vi "Unpack for gRPC.vi"(8 "error in":errorcluster, 9 "configuration / results":enum16{"Configuration", "Results"}(ring), 10 "any":T1, 11 "measurement plugin in":refnum<class "Automotive Vision.lvclass">) -> (0 "error out":errorcluster, 2 "data value":variant, 3 "measurement plugin out":refnum<class "Automotive Vision.lvclass">)   [LabVIEW 2025, in "Automotive Vision.lvclass"]
uses:
  Automotive Vision.lvclass
  <vilib>/gRPC/LabVIEW gRPC Library/Shared/Any.ctl
  C:/Program Files/National Instruments/LabVIEW 2025/vi.lib/Plug-In SDKs/Measurements/Measurement Plugin Service/Measurement Plugin Service.lvclass
  Measurement Configuration.ctl
  Measurement Results.ctl
  a521b266-ce99-437c-923d-067dcf1e07fd.vi
  3ecd018e-d556-4cbc-bc60-c4ba57204520.vi
  <vilib>/gRPC/LabVIEW gRPC Library/Server API/Translate Protobuf Error.vi
  <vilib>/AdvancedString/1D String Array to Delimited String.vi
  <vilib>/gRPC/LabVIEW gRPC Library/Server API/Server/Get Server DLL Path.vi
  <vilib>/Plug-In SDKs/Measurements/Measurement Plugin Service/Measurement Plugin Service.lvclass
  <vilib>/gRPC/LabVIEW gRPC Library/grpc-lvsupport-release.lvlib
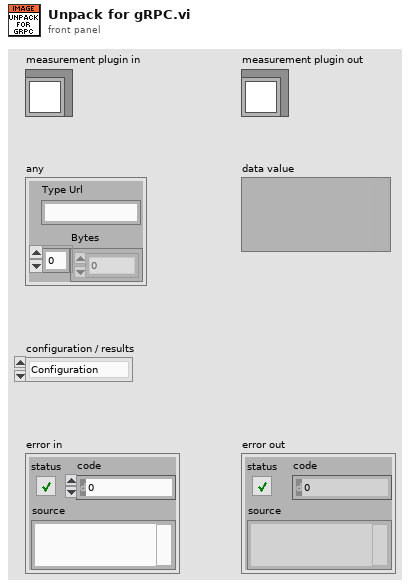
[diagram p1: front panel]
types:
  T1 = typedef "grpc-lvsupport-release.lvlib/Any.ctl" = cluster{"Type Url":string, "Bytes":u8[]}
  T2 = typedef "grpc-lvsupport-release.lvlib/grpcId.ctl" = u64
  T3 = typedef "Automotive Vision.lvclass/Measurement Configuration.ctl" = cluster{"SERIAL CHANNEL":string, "PATH TO CONFIGURATION SCRIPT":string, "REF. CLOCK  (Hz)":dbl, "POC SOURCE":u32, "CSI-2 DATA SOURCE":u32, "SI ACTIVE LANE CNT":u32, "PAYLOAD DATA TYPE":enum32{"Frame Start", "Frame End", "Line Start", "Line End", "End of Transmission", "Reserved 0", "Reserved 1", "Reserved 2", "Generic Short Packet 1", "Generic Short Packet 2", "Generic Short Packet 3", "Generic Short Packet 4", "Generic Short Packet 5", "Generic Short Packet 6", "Generic Short Packet 7", "Generic Short Packet 8", "Null", "Blanking Data", "Embedded 8-bit non Image Data", "Generic Long Packet 1", "Generic Long Packet 2", "Generic Long Packet 3", "Generic Long Packet 4", "Reserved 3", "YUV420 8-bit", "YUV420 10-bit", "Legacy YUV420 8-bit", "Reserved 4", "YUV420 8-bit Chroma Shifted", "YUV420 10-bit Chroma Shifted", "YUV422 8-bit", "YUV422 10-bit", "RGB444", "RGB555", "RGB565", "RGB666", "RGB888", "Reserved 5", "Reserved 6", "RAW 24", "RAW 6", "RAW 7", "RAW 8", "RAW 10", "RAW 12", "RAW 14", "RAW 16", "RAW 20", "User Defined 8-bit Data 1", "User Defined 8-bit Data 2", "User Defined 8-bit Data 3", "User Defined 8-bit Data 4", "User Defined 8-bit Data 5", "User Defined 8-bit Data 6", "User Defined 8-bit Data 7", "User Defined 8-bit Data 8", "USL Command", "Reserved 7", "Reserved 8", "Reserved 9", "Reserved 10", "Reserved 11", "Reserved 12", "LRTE EPD Spacer"}, "INTERPRETATION":u32, "VIRTUAL CHANNEL":u32, "PATTERN":u32, "ALGORITHM":u32, "RIO HANDLER":string, "AUTO. VISION DEVICE":u32, "SERIAL (SI) CHANNEL":u32, "BITFILE":string}
  T4 = typedef "Automotive Vision.lvclass/Measurement Results.ctl" = cluster{"ACQ. IN PROGRESS":bool, "IMAGE PIXEL DATA":u32[], "ACQ. DURATION (s)":dbl, "SOURCE RATE (fps)":dbl, "BYTES ACQUIRED":u64, "FRAME COUNT":u64, "POC VOLTAGE (V)":dbl, "POC CURRENT (A)":dbl, "ERROR":bool, "STATE MESSAGE":string, "IMAGE DATA":string, "OOB gRPC Port":i32, "HEIGHT":u64, "WIDTH":u64}
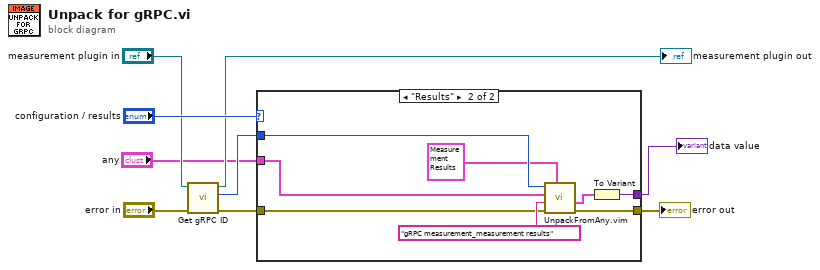
[diagram p0: block diagram]
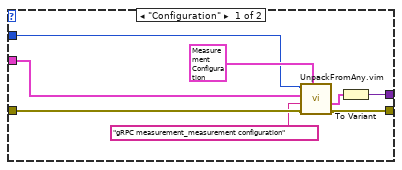
[diagram p2: hidden frame]
diagram:
  n1 = call <vilib>:"Get gRPC ID.vi"("error in"="error in", "measurement plugin service in"="measurement plugin in") -> ("error out"=w6:errorcluster, "gRPC ID"=w3:T2, "measurement plugin service out"=→"measurement plugin out":refnum<class "Automotive Vision.lvclass">)  [unwired: 7 in]
  n2 = case shown="\"Results\"" "configuration / results" {
    tunnel: w6 -> [w15 w19]
    tunnel: "any" -> [w10 w18]
    tunnel: w3 -> [w12 w22]
    tunnel: [w16 w23] -> w9
    tunnel: [w17 w25] -> w1
    frame "Configuration" {
      n3 = call "UnpackFromAny.vim"("Data Type"=T3 {"SERIAL CHANNEL"="Lorem ipsum dolor sit", "PATH TO CONFIGURATION SCRIPT"="", "REF. CLOCK  (Hz)"=1.2, "POC SOURCE"=32, "CSI-2 DATA SOURCE"=1, "SI ACTIVE LANE CNT"=1, "PAYLOAD DATA TYPE"=enum."Frame Start", "INTERPRETATION"=0, "VIRTUAL CHANNEL"=0, "PATTERN"=0, "ALGORITHM"=0, "RIO HANDLER"="", "AUTO. VISION DEVICE"=0, "SERIAL (SI) CHANNEL"=0, "BITFILE"="IMAGE RESOLUTION: 800x600 - RAW12"} ("Measurement Configuration"), "error in"=w15, "Message Type"="gRPC measurement_measurement configuration", "Any"=w10, "gRPCid in"=w12) -> ("error out"=w16:errorcluster, "Unpacked Value"=w14:T3)  [unwired: 4 in, 1 out]
      n4 = To Variant(anything=w14) -> (Variant=w17:variant)
    }
    frame "Results" {
      n5 = call "UnpackFromAny.vim"("Data Type"=T4 {"ACQ. IN PROGRESS"=FALSE, "IMAGE PIXEL DATA"=[], "ACQ. DURATION (s)"=0.0, "SOURCE RATE (fps)"=0.0, "BYTES ACQUIRED"=0, "FRAME COUNT"=0, "POC VOLTAGE (V)"=0.0, "POC CURRENT (A)"=0.0, "ERROR"=FALSE, "STATE MESSAGE"="", "IMAGE DATA"="", "OOB gRPC Port"=0, "HEIGHT"=0, "WIDTH"=0} ("Measurement Results"), "error in"=w19, "Message Type"="gRPC measurement_measurement results", "Any"=w18, "gRPCid in"=w22) -> ("error out"=w23:errorcluster, "Unpacked Value"=w24:T4)  [unwired: 4 in, 1 out]
      n6 = To Variant(anything=w24) -> (Variant=w25:variant)
    }
  }
  "error out" <- w9
  "data value" <- w1
